vi "Binary Morphological Reconstruction - Find Particle.vi"() -> ()   [LabVIEW 2014]
doc: "This example demonstrates a binary morphological reconstruction to find the objects thicker than the specified value. First, a distance transform is applied to the source image. Next, image is thresholded using the Minimum width. The Binary Morphological reconstruction is applied to the resulting image to get objects thicker than the specified value."
uses:
  <vilib>/vision/NI_Vision_Development_Module.lvlib
panel:
  in  "Images":T1(tab)=enum."5. Morphological Reconstruction"
  out "Source Image":T2(plugin-control)
  out "Threshold Image":T2(plugin-control)
  out "Distance Image":T2(plugin-control)
  out "Threshold Distance":T2(plugin-control)
  out "Reconstructed Image":T2(plugin-control)
  # "Overview: Demonstrate the use of the binary morphological reconstruction feature of Vision Development Module.\nThis example thresholds an image, computes the distance, and reconstructs only objects whose width is greater than the number specified.\nRequirements: Vision Development Module.\nInstructions:\n1. Run the VI.\n2. Select the different tabs to view the image corresponding to each of the functions."
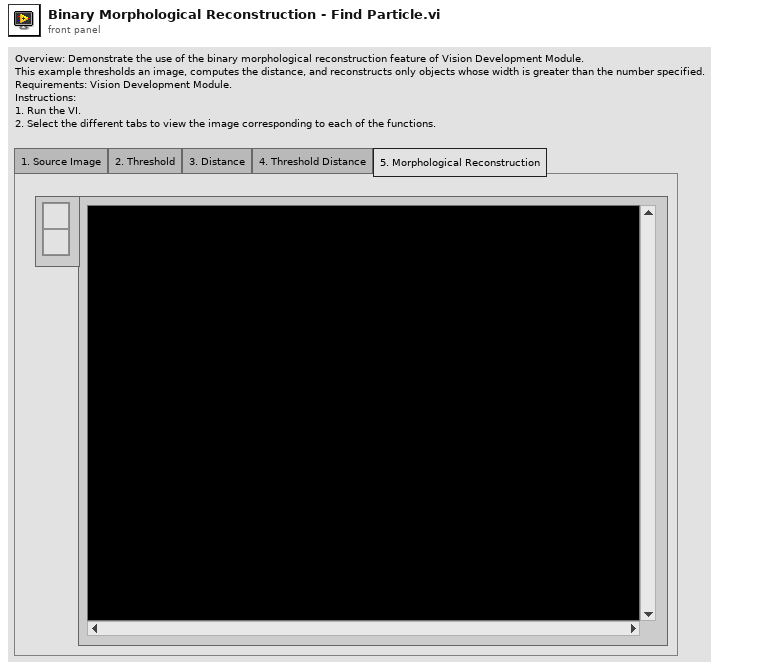
[diagram p1: front panel]
types:
  T1 = enum32{"1. Source Image", "2. Threshold", "3. Distance", "4. Threshold Distance", "5. Morphological Reconstruction"}
  T2 = typedef "IMAQ Image.ctl" = refnum<image>
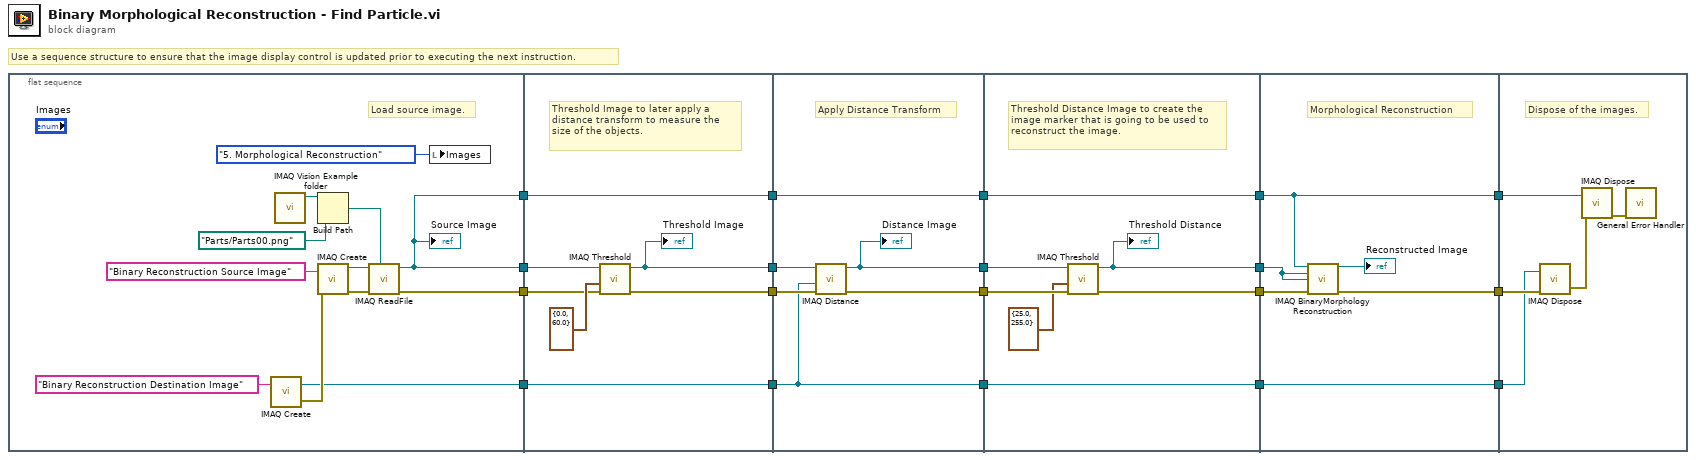
[diagram p0: block diagram]
diagram:
  # "Use a sequence structure to ensure that the image display control is updated prior to executing the next instruction."
  n1 = flat-sequence {
    tunnel: [w27] -> w19
    tunnel: [w23] -> w18
    tunnel: [w24] -> w17
    tunnel: [w23] -> w7
    tunnel: w19 -> [w36]
    tunnel: w18 -> [w37]
    tunnel: w17 -> [w33]
    tunnel: [w35] -> w16
    tunnel: [w34] -> w15
    tunnel: [w33] -> w12
    tunnel: [w32] -> w8
    tunnel: w7 -> [w32]
    tunnel: w16 -> [w43]
    tunnel: w15 -> [w44]
    tunnel: [w42] -> w14
    tunnel: [w41] -> w13
    tunnel: w12 -> [w39]
    tunnel: [w40] -> w9
    tunnel: w8 -> [w40]
    tunnel: [w39] -> w1
    tunnel: w14 -> [w51]
    tunnel: w13 -> [w50]
    tunnel: [w49] -> w11
    tunnel: [w48] -> w10
    tunnel: w9 -> [w48]
    tunnel: [w47] -> w6
    tunnel: [w46] -> w2
    tunnel: w1 -> [w46]
    tunnel: w11 -> [w57]
    tunnel: w10 -> [w53]
    tunnel: w6 -> [w55]
    tunnel: [w54] -> w5
    tunnel: [w53] -> w4
    tunnel: [w52] -> w3
    tunnel: w2 -> [w52]
    tunnel: w5 -> [w62]
    tunnel: w4 -> [w61]
    tunnel: w3 -> [w58]
    frame #0 {
      # "Load source image."
      n2 = call "IMAQ Create"("Image Name"="Binary Reconstruction Destination Image") -> ("New Image"=w24:T2, "error out"=w25:errorcluster)  [unwired: 3 in, 1 out]
      n3 = call "IMAQ Vision Example folder.vi"() -> ("Example Image Path"=w30:path)  [unwired: 11 in]
      n4 = Build Path(base path=w30, name or relative path=path "Parts/Parts00.png" ("appended path")) -> (appended path=w22:path)
      n5 = call "IMAQ Create"("Image Name"="Binary Reconstruction Source Image", "error in (no error)"=w25) -> ("New Image"=w29:T2, "error out"=w28:errorcluster)  [unwired: 2 in, 1 out]
      n6 = call "IMAQ ReadFile"("File Path"=w22, "error in (no error)"=w28, "Image"=w29) -> ("error out"=w27:errorcluster, "Image Out"=w23:T2)  [unwired: 2 in, 5 out]
      "Source Image" <- w23
      n7 = local write "Images"(T1."5. Morphological Reconstruction" ("Images")) -> ()
    }
    frame #1 {
      # "Threshold Image to later apply a distance transform to measure the size of the objects."
      n8 = call "IMAQ Threshold"("error in (no error)"=w36, "Range"=cluster{"Lower value":sgl, "Upper value":sgl} {"Lower value"=0.0, "Upper value"=60.0}, "Image Src"=w37) -> ("error out"=w35:errorcluster, "Image Dst Out"=w34:T2)  [unwired: 3 in, 4 out]
      "Threshold Image" <- w34
    }
    frame #2 {
      # "Apply Distance Transform"
      n9 = call "IMAQ Distance"("error in (no error)"=w43, "Image Dst"=w39, "Image Src"=w44) -> ("error out"=w41:errorcluster, "Image Dst Out"=w42:T2)  [unwired: 1 in, 2 out]
      "Distance Image" <- w42
    }
    frame #3 {
      # "Threshold Distance Image to create the image marker that is going to be used to reconstruct the image."
      n10 = call "IMAQ Threshold"("error in (no error)"=w50, "Range"=cluster{"y":sgl, "Upper value":sgl} {"y"=25.0, "Upper value"=255.0} ("output cluster"), "Image Src"=w51) -> ("error out"=w47:errorcluster, "Image Dst Out"=w49:T2)  [unwired: 3 in, 4 out]
      "Threshold Distance" <- w49
    }
    frame #4 {
      # "Morphological Reconstruction"
      n11 = call "IMAQ BinaryMorphology Reconstruction"("Image Src"=w53, "Image Dst"=w57, "Image Marker"=w57, "error in (no error)"=w55) -> ("Image Dst Out"=→"Reconstructed Image":T2, "error out"=w54:errorcluster)  [unwired: 4 in, 6 out]
    }
    frame #5 {
      # "Dispose of the images."
      n12 = call "IMAQ Dispose"("Image"=w58, "error in (no error)"=w62) -> ("error out"=w60:errorcluster)  [unwired: 1 in, 3 out]
      n13 = call "IMAQ Dispose"("Image"=w61, "error in (no error)"=w60) -> ("error out"=w59:errorcluster)  [unwired: 1 in, 3 out]
      n14 = call <vilib>:"General Error Handler.vi"("error in (no error)"=w59) -> ()  [unwired: 10 in, 5 out]
    }
  }
